vi "run sipper pump manual.vi"(3 "GPIB in":string="18") -> ()   [LabVIEW 2015]
panel:
  in  "done":bool
  # "Pump is running. Pump will\nstop when you press OK."
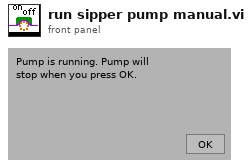
[diagram p1: front panel]
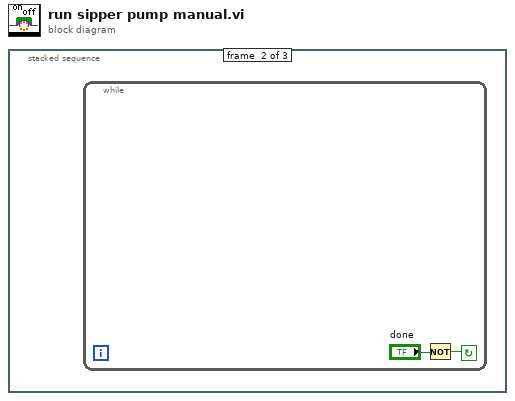
[diagram p0: block diagram]
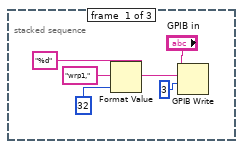
[diagram p2: hidden frame]
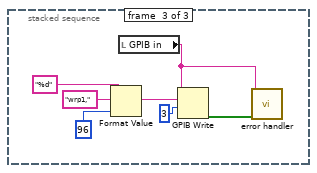
[diagram p3: hidden frame]
diagram:
  n1 = stacked-sequence {
    frame #0 {
      n2 = Format Value(string ("")="wrp1,", format string="%d", value (0)=32) -> (output string=w5:string)
      n3 = GPIB Write(0:"GPIB in", 1:w5, 2:3) -> ()  [unwired: 2 in, 2 out]
    }
    frame #1 {
      n4 = while {
        stop <- w7 continue-if-true
        n5 = Not(x="done") -> (.not. x?=w7:bool)
      }
    }
    frame #2 {
      n6 = Format Value(string ("")="wrp1,", format string="%d", value (0)=96) -> (output string=w13:string)
      n7 = local read "GPIB in"() -> (w9:string)
      n8 = GPIB Write(0:w9, 1:w13, 2:3) -> (5:w15:bool[])  [unwired: 2 in, 1 out]
      n9 = call "error handler.vi"("status array"=w15, "GPIB in"=w9) -> ()  [unwired: 3 in, 3 out]
    }
  }
